vi "MainRT_APA_BACK_221005.vi"() -> ()   [LabVIEW 2019]
uses:
  <vilib>/myRIO/Instrument Drivers/Onboard IO/UART/typedef/VISA Configuration.ctl
  <vilib>/Platform/TimedLoop/XDataNode/timing_clust.ctl
  <vilib>/Platform/TimedLoop/XDataNode/nitl_modes.ctl
  <vilib>/Platform/TimedLoop/XDataNode/wakeup.ctl
  <vilib>/FPGAPlugInAG/myRIO-1900/niLvFpga_Open_myRIO-1900.vi
  <vilib>/rvi/interface/common/dynamic/niFpgaDynamicAddResources.vi
  <vilib>/Utility/error.llb/Error Cluster From Error Code.vi
  <vilib>/rvi/errors/niLvFpgaAdjustHostInterfaceError.vi
  <vilib>/FPGAPlugInAG/Dynamic/niLvFpga_Close_Dynamic.vi
  <vilib>/platform/TimedLoop/XDataNode/XDataNode.xnode
  <vilib>/rvi/interface/nirviOpenFPGA/nirviOpenFPGA.xnode
  FPGA Bitfiles/apa_FPGATarget_MainFPGAAPA_997zCpBZn8o.lvbitx
  MainFPGA_APA.vi
  <vilib>/rvi/interface/nirviReadWriteControl/nirviReadWriteControl.xnode
  <vilib>/rvi/interface/nirviCloseFPGA/nirviCloseFPGA.xnode
  <vilib>/Instr/_visa.llb/VISA Configure Serial Port (Instr).vi
  <vilib>/Platform/TimedLoop/XDataNode/XDNodeRunTimeDep.lvlib
  <vilib>/myRIO/Instrument Drivers/Onboard IO/UART/UART.lvlib
  NiFpgaLv.dll
  <vilib>/rvi/interface/Simulation/niFpgaSimulationCallBeginRW.vi
panel:
  out "Waveform Chart":cluster{"Gyro_z":dbl, dbl}(graph)
  out "Gyro_z":dbl
  in  "Period":i64=1
  out "Latency":i16
  in  "error in":errorcluster
  in  "file no.":u32
  out "error out":errorcluster
  in  "stop":bool
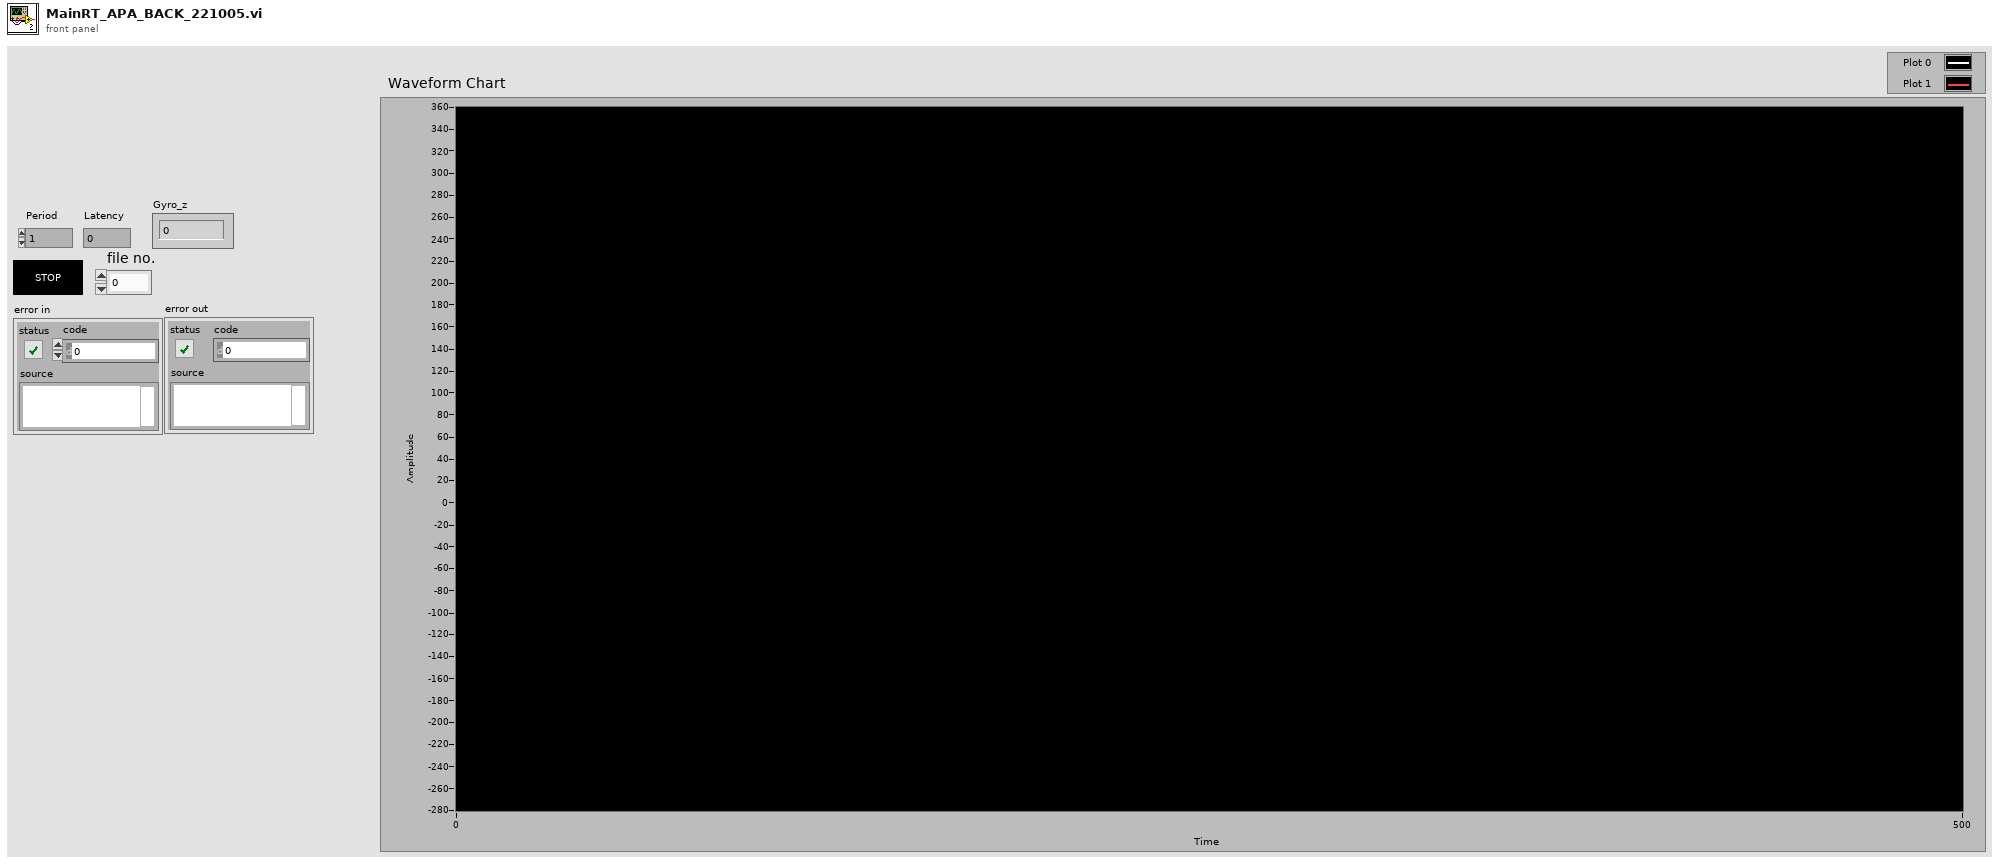
[diagram p1: front panel]
types:
  T1 = typedef "UART.lvlib/VISA Configuration.ctl" = cluster{"baud rate (9600)":u32, "data bits (8)":u16, "parity (0:none)":enum16{"None", "Odd", "Even", "Mark", "Space"}, "stop bits (10: 1 bit)":u16, "flow control (0:none)":u16, "termination char\n(0xA = '\\n' = LF) ":u8, "Enable Termination\nChar (T)":bool, "timeout (10sec)":u32}
  T2 = enum16{"open", "replace", "create", "open or create", "replace or create", "replace or create with confirmation"}
  T3 = typedef "XDNodeRunTimeDep.lvlib/timing_clust.ctl" = cluster{"Expected End [f-1]":u64, "Actual End [f-1]":u64, "Finished Late? [f-1]":bool, "Expected End [i-1]":u64, "Actual End [i-1]":u64, "Finished Late? [i-1]":bool, "Expected Start [i]":u64, "Actual Start [i]":u64, "Expected Start [f]":u64, "Actual Start [f]":u64, "Source Name":string, "Structure Name":string, "Period":i64, "Deadline":i64, "Offset":i64, "Start":i64, "Priority":i32, "Timeout":i32, "Mode":T4, "Wakeup Reason":T5, "Error":errorcluster, "Source Type":string, "Secondary Source Type":string, "Global End Time":u64, "Global Start Time":u64, "Frame Duration":u64, "Iteration Duration":u64, "Assigned CPU":i32, "I/O Scan Engine Mode":u32}
  T4 = typedef "XDNodeRunTimeDep.lvlib/nitl_modes.ctl" = enum32{"No Change", "Process missed periods, maintain original phase", "Discard missed periods, maintain original phase", "Process missed periods, ignore original phase", "Discard missed periods, ignore original phase"}
  T5 = typedef "XDNodeRunTimeDep.lvlib/wakeup.ctl" = enum32{"Normal", "Aborted", "Asynchronous wakeup", "Timing source error", "Timed loop error", "Timeout"}
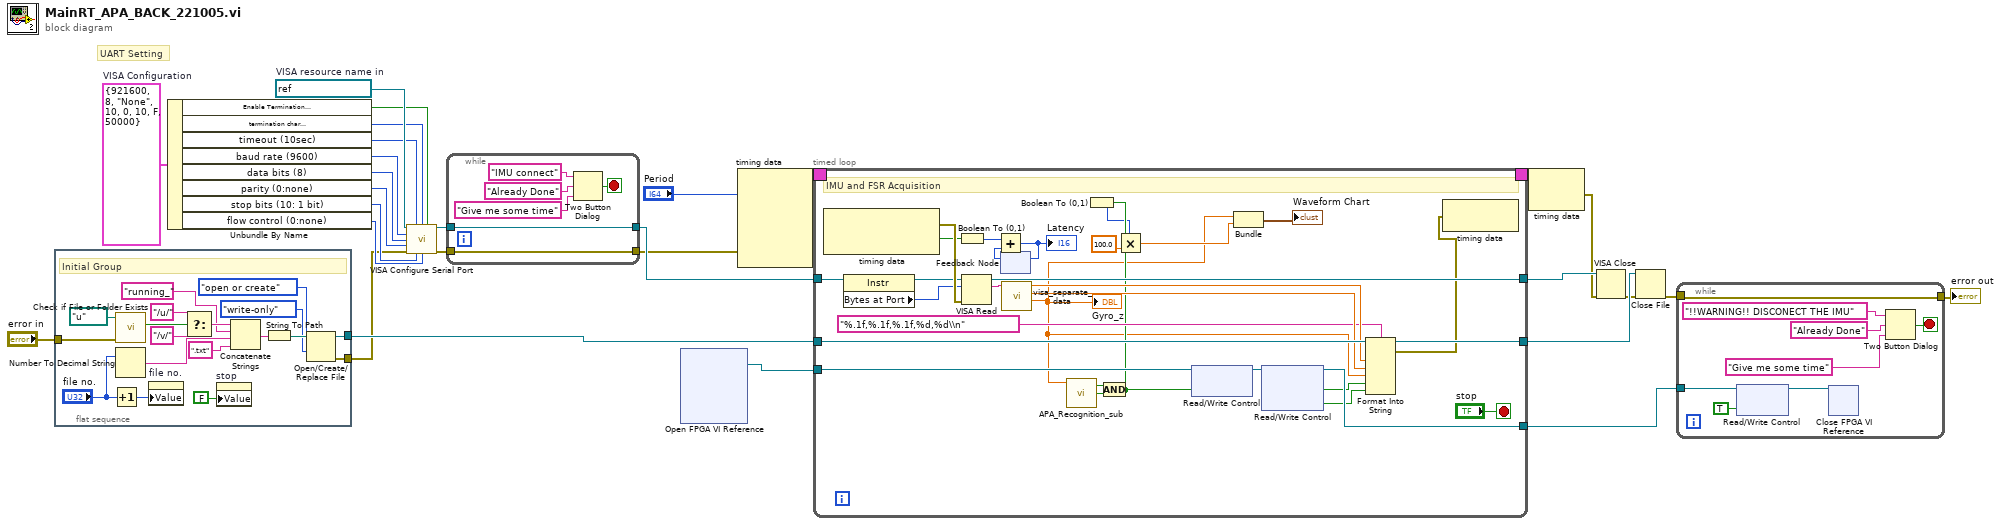
[diagram p0: block diagram]
diagram:
  w25 = T1 {"baud rate (9600)"=921600, "data bits (8)"=8, "parity (0:none)"=enum."None", "stop bits (10: 1 bit)"=10, "flow control (0:none)"=0, "termination char\n(0xA = '\\n' = LF) "=10, "Enable Termination\nChar (T)"=FALSE, "timeout (10sec)"=50000}  # VISA Configuration
  w26 = refnum<visa-resource-name> "ASRL1::INSTR"  # VISA resource name in
  # "UART Setting"
  n1 = flat-sequence {
    tunnel: "error in" -> [w30]
    tunnel: [w31] -> w5
    tunnel: [w29] -> w4
    frame #0 {
      # "Initial Group"
      n2 = Increment(x="file no.") -> (x+1=w44:u32)
      n3 = call <vilib>:"Check if File or Folder Exists.vi"("error in (no error)"=w30, "path"=path "u:/") -> ("file or folder exists?"=w39:bool)  [unwired: 7 in, 2 out]
      n4 = Number To Decimal String(number="file no.") -> (decimal integer string=w43:string)  [unwired: 1 in]
      n5 = property on="file no." class="DigNum (strict)"("Value"=w44) -> ()  [unwired: 2 in, 2 out]
      n6 = Select(t="/u/", s=w39, f="/v/") -> (s? t:f=w41:string)
      n7 = property on="stop" class="Bool (strict)"("Value"=FALSE ("stop")) -> ()  [unwired: 2 in, 2 out]
      n8 = Concatenate Strings(w41, "running_" ("string"), w43, ".txt" ("string")) -> (w42:string)
      n9 = String To Path(string=w42) -> (path=w40:path)
      n10 = Open/Create/Replace File(file path (use dialog)=w40, operation (0:open)=T2."open or create", access (0:read/write)=enum16{"read/write", "read-only", "write-only"}."write-only") -> (refnum out=w31:refnum<file>, error out=w29:errorcluster)  [unwired: 3 in, 1 out]
    }
  }
  n11 = Unbundle By Name(w25) -> ("Enable Termination\nChar (T)"=w24:bool, "termination char\n(0xA = '\\n' = LF)"=w23:u8, "timeout (10sec)"=w22:u32, "baud rate (9600)"=w18:u32, "data bits (8)"=w19:u16, "parity (0:none)"=w20:enum16{"None", "Odd", "Even", "Mark", "Space"}, "stop bits (10: 1 bit)"=w21:u16, "flow control (0:none)"=w17:u16)
  n12 = call-poly "VISA Configure Serial Port"("VISA resource name"=w26, "timeout (10sec)"=w22, "termination char\n(0xA = '\\n' = LF)"=w23, "Enable Termination\nChar (T)"=w24, "baud rate (9600)"=w18, "data bits (8)"=w19, "parity (0:none)"=w20, "error in (no error)"=w4, "stop bits (10: 1 bit)"=w21, "flow control (0:none)"=w17) -> ("VISA resource name out"=w14:refnum<visa-resource-name>, "error out"=w13:errorcluster)  [unwired: 4 in]
  n13 = while {
    tunnel: [w52] -> w10
    tunnel: w13 -> [w52]
    tunnel: [w51] -> w12
    tunnel: w14 -> [w51]
    stop <- w47 stop-if-true
    n14 = Two Button Dialog(message="IMU connect", 1:"Give me some time" ("F button name (\"Cancel\")"), 2:"Already Done" ("button name (\"OK\")")) -> (T button?=w47:bool)
  }
  n15 = xnode ("Open FPGA VI Reference")() -> ("FPGA VI Reference Out"=w9:refnum<k20>)  [unwired: 2 in, 1 out]
  n16 = node-c288("Period", w10) -> (w28:T3)  [unwired: 3 in]
  n17 = timed-loop {
    timing: w28 -> [_]
    timing-out: [_] -> w27
    tunnel: w12 -> [w78]
    tunnel: [w82] -> w16
    tunnel: w9 -> [w62]
    tunnel: [w72] -> w3
    tunnel: w5 -> [w75]
    tunnel: [w74] -> w8
    stop <- "stop" stop-if-true
    # "IMU and FSR Acquisition"
    n18 = node-c288() -> (w80:errorcluster, w66:bool)  [unwired: 1 in]
    n19 = property class="Instr"(reference=w78) -> (reference out=w77:refnum<visa-resource-name>, "Bytes at Port"=w76:u32)  [unwired: 1 in, 1 out]
    n20 = Boolean To (0,1)(Boolean=w66) -> (0, 1=w65:i16)
    n21 = VISA Read(VISA resource name=w77, byte count=w76, error in (no error)=w80) -> (VISA resource name out=w82:refnum<visa-resource-name>, read buffer=w81:string)  [unwired: 2 out]
    n22 = feedback #1() -> (w63:i16)  [unwired: 1 in]
    n23 = Add(x=w65, y=w63) -> (x+y=w64:i16)
    "Latency" <- w64
    n24 = feedback-in #1(w64) -> ()
    n25 = call "visa_separate_data.vi"("Input string"=w81) -> ("Gyro_z"=w53:dbl, "Gyro_y"=w69:dbl, "Gyro_x"=w70:dbl)  [unwired: 7 in, 1 out]
    "Gyro_z" <- w53
    n26 = call "APA_Recognition_sub.vi"("IMU_IN[k]"=w53) -> ("Same Sagittal Direction"=w60:bool, "Assist Reference"=w61:bool)  [unwired: 8 in, 1 out]
    n27 = And(x=w61, y=w60) -> (x .and. y?=w58:bool)
    n28 = Boolean To (0,1)(Boolean=w58) -> (0, 1=w56:i16)
    n29 = Multiply(x=w56, y=100.0) -> (x*y=w55:dbl)
    n30 = xnode "Read/Write Control"("FPGA VI Reference In"=w62, "A_Digit0"=w58) -> ("FPGA VI Reference Out"=w71:refnum<k20>)  [unwired: 1 in, 1 out]
    n31 = Bundle("Gyro_z"=w53, w55) -> (→"Waveform Chart":cluster{"Gyro_z":dbl, dbl})  [unwired: 1 in]
    n32 = xnode "Read/Write Control"("FPGA VI Reference In"=w71) -> ("FPGA VI Reference Out"=w72:refnum<k20>, "A_Digit0"=w59:bool, "A_Digit3"=w68:bool)  [unwired: 1 in, 1 out]
    n33 = Format Into String(format string="%.1f,%.1f,%.1f,%d,%d\\n", initial string=w75, w70, w69, w53, w59, w68) -> (resulting string=w74:refnum<file>, error out=w73:errorcluster)  [unwired: 1 in]
    n34 = node-c288(w73) -> ()  [unwired: 1 out]
  }
  n35 = node-c288(w27) -> (w7:errorcluster)
  n36 = VISA Close(VISA resource name=w16, error in (no error)=w7) -> (error out=w6:errorcluster)
  n37 = Close File(refnum=w8, error in=w6) -> (error out=w2:errorcluster)  [unwired: 1 out]
  n38 = while {
    tunnel: [w96] -> w15
    tunnel: w2 -> [w96]
    tunnel: w3 -> [w91]
    stop <- w92 stop-if-true
    n39 = xnode "Read/Write Control"("FPGA VI Reference In"=w91, "stop"=TRUE) -> ("FPGA VI Reference Out"=w89:refnum<k20>)  [unwired: 1 in, 1 out]
    n40 = xnode "Close FPGA VI Reference"("FPGA VI Reference In"=w89) -> ()  [unwired: 1 in, 1 out]
    n41 = Two Button Dialog(message="!!WARNING!! DISCONECT THE IMU", 1:"Give me some time" ("F button name (\"Cancel\")"), 2:"Already Done" ("button name (\"OK\")")) -> (T button?=w92:bool)
  }
  "error out" <- w15
